vi "UTILITY Counter.vi"(4 "Reset":bool) -> (0 "Count":dbl)   [LabVIEW 2018]
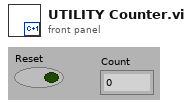
[diagram p1: front panel]
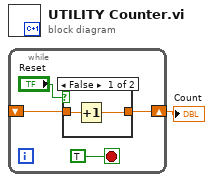
[diagram p0: block diagram]
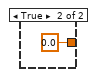
[diagram p2: hidden frame]
diagram:
  n1 = while {
    shift-right: [w4] -> w1
    shift-left: _ -> [w3]
    stop <- TRUE stop-if-true
    n2 = case shown="False" "Reset" {
      tunnel: [w7 0.0] -> w4
      tunnel: w3 -> [w6 _]
      frame False {
        n3 = Increment(x=w6) -> (x+1=w7:dbl)
      }
      frame True {
      }
    }
  }
  "Count" <- w1
